vi "Test Disconnection by Peer Errors.vi"() -> ()   [LabVIEW 2013]
uses:
  source/MQTT_Connection/Connection/Connection.lvclass
panel:
  out "error out 3":errorcluster
  out "error out 2":errorcluster
  out "error out":errorcluster
  out "error out 9":errorcluster
  out "error out 8":errorcluster
  out "error out 7":errorcluster
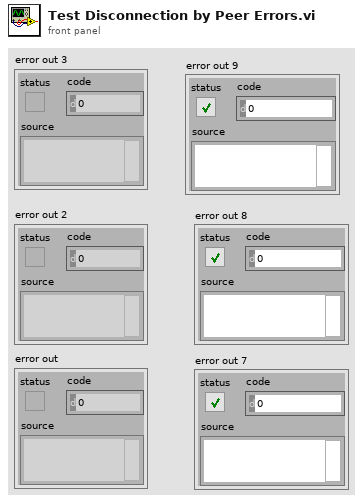
[diagram p1: front panel]
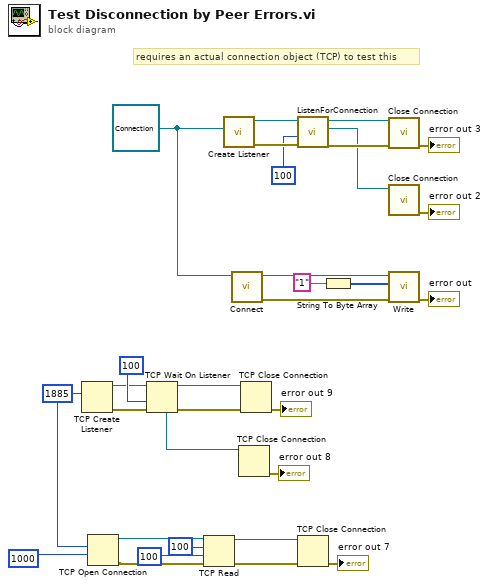
[diagram p0: block diagram]
diagram:
  w19 = u16 1885 ("port")
  w16 = refnum<class "Connection.lvclass"> refnum ("MQTT_Connection.lvlib:Connection.lvclass")
  # "requires an actual connection object (TCP) to test this"
  n1 = TCP Create Listener(10:w19) -> (0:w23:errorcluster, 3:w20:refnum<k5>)  [unwired: 4 in, 1 out]
  n2 = TCP Open Connection(remote port or service name=w19, timeout ms (60000)=1000 ("timeout ms (wait forever: -1)")) -> (connection ID=w9:refnum<k5>, error out=w8:errorcluster)  [unwired: 3 in]
  n3 = TCP Wait On Listener(8:w23, 9:100 ("timeout ms (wait forever: -1)"), 11:w20) -> (0:w24:errorcluster, 3:w22:refnum<k5>, 4:w18:refnum<k5>)  [unwired: 1 in, 2 out]
  n4 = TCP Read(connection ID=w9, bytes to read=100, error in (no error)=w8, 9:100 ("bytes to read")) -> (connection ID out=w5:refnum<k5>, error out=w4:errorcluster)  [unwired: 1 in, 1 out]
  n5 = call "Create Listener.vi"("Connection Configuration"=w16) -> ("error out"=w28:errorcluster, "Listener"=w31:refnum<class "Connection.lvclass">)  [unwired: 9 in]
  n6 = call "Connect.vi"("Connection in"=w16) -> ("error out"=w1:errorcluster, "Connection out"=w15:refnum<class "Connection.lvclass">)  [unwired: 9 in]
  n7 = TCP Close Connection(connection ID=w18) -> (error out=→"error out 8":errorcluster)  [unwired: 2 in, 1 out]
  n8 = TCP Close Connection(connection ID=w22, error in (no error)=w24) -> (error out=→"error out 9":errorcluster)  [unwired: 1 in, 1 out]
  n9 = call "ListenForConnection.vi"("error in (no error)"=w28, "timeout (2000 ms)"=100 ("timeout ms (wait forever: -1)"), "Listener"=w31) -> ("error out"=w29:errorcluster, "Connection"=w14:refnum<class "Connection.lvclass">, "Listener out"=w30:refnum<class "Connection.lvclass">)  [unwired: 5 in, 1 out]
  n10 = TCP Close Connection(connection ID=w5, error in (no error)=w4) -> (error out=→"error out 7":errorcluster)  [unwired: 1 in, 1 out]
  n11 = String To Byte Array(string="1" ("data in")) -> (unsigned byte array=w26:u8[])
  n12 = call "Close Connection.vi"("error in (no error)"=w29, "Connection in"=w30) -> ("error out"=→"error out 3":errorcluster)  [unwired: 8 in, 1 out]
  n13 = call "Close Connection.vi"("Connection in"=w14) -> ("error out"=→"error out 2":errorcluster)  [unwired: 9 in, 1 out]
  n14 = call "Write.vi"("error in (no error)"=w1, "Bytes"=w26, "Connection in"=w15) -> ("error out"=→"error out":errorcluster)  [unwired: 7 in, 1 out]
